vi "Autonomous Independent.vi"   [LabVIEW 2016]
doc: "This VI is called when autonomous begins, and will automatically be terminated when autonomous ends. You can carry out timed or sensor driven robot movement independently without needing to return to the caller."
uses:
  <vilib>/Rock Robotics/WPI/Utilities/WPI_GetSetVariantRefNum.vi
  <vilib>/Rock Robotics/Network Tables/NT Read String.vi
  <vilib>/Rock Robotics/Network Tables/NT Write Numeric Array.vi
  Robot Global Data.vi
  <vilib>/addons/control/pid/pid.llb/PID (DBL).vi
  <vilib>/addons/control/pid/NI_PID_pid.lvlib
panel:
  # "Be sure to right-click and choose Data Operations>>Make Current Value default if you want to save the array values with the VI"
types:
  T1 = typedef "WPI_JoystickDevRef.ctl" = cluster{"Device":T2}
  T2 = typedef "WPI_JoystickDeviceEnum.ctl" = enum16{"USB 0", "USB 1", "USB 2", "USB 3", "USB 4", "USB 5"}
  T3 = typedef "WPI_RobotDriveDevRef.ctl" = cluster{"DevStatus":errorcluster, "Motors[]":T4[], "Square Inputs":bool, "Max Output":dbl}
  T4 = typedef "WPI_MotorControlDeviceRef.ctl" = cluster{"DeviceStatus":errorcluster, "Type":T5, "PWM":cluster{"PWM Channel":T6, "DeadBand":T7}, "CAN":cluster{"Device Number":u8, "SetOutput VI Ref":variant, "GetOutput VI Ref":variant, "Enable VI Ref":variant, "Disable VI Ref":variant, "Data":variant}, "Invert":bool}
  T5 = typedef "WPI_MotorControlType.ctl" = enum16{"PWM", "CAN"}
  T6 = typedef "FPGA_DIOPWMChannel.ctl" = enum8{"PWM 0", "PWM 1", "PWM 2", "PWM 3", "PWM 4", "PWM 5", "PWM 6", "PWM 7", "PWM 8", "PWM 9", "PWM MXP 0", "PWM MXP 1", "PWM MXP 2", "PWM MXP 3", "PWM MXP 4", "PWM MXP 5", "PWM MXP 6", "PWM MXP 7", "PWM MXP 8", "PWM MXP 9", "Invalid"}
  T7 = typedef "WPI_PWMDeadband.ctl" = cluster{"Name":string, "maxPositivePwm":i32, "minPositivePwm":i32, "centerPwm":i32, "maxNegativePwm":i32, "minNegativePwm":i32, "angularRange":u16}
  T8 = cluster{"proportional gain (Kc)":dbl, "integral time (Ti, min)":dbl, "derivative time (Td, min)":dbl}
  T9 = cluster{"Distance (ft)":dbl, "Score":dbl, "Normalized":cluster{"Center":cluster{dbl, dbl}, "Rectangle":cluster{"Numeric":dbl, "Numeric 2":dbl, "Numeric 3":dbl, "Numeric 5":dbl}}, "Pixels":cluster{"Center":cluster{dbl, dbl}, "Rectangle":cluster{"Numeric":dbl, "Numeric 2":dbl, "Numeric 3":dbl, "Numeric 5":dbl}}}
  T10 = cluster{"Yaw":dbl, "Roll":dbl, "Pitch":dbl, "Heading":dbl, "Fused Heading":dbl}
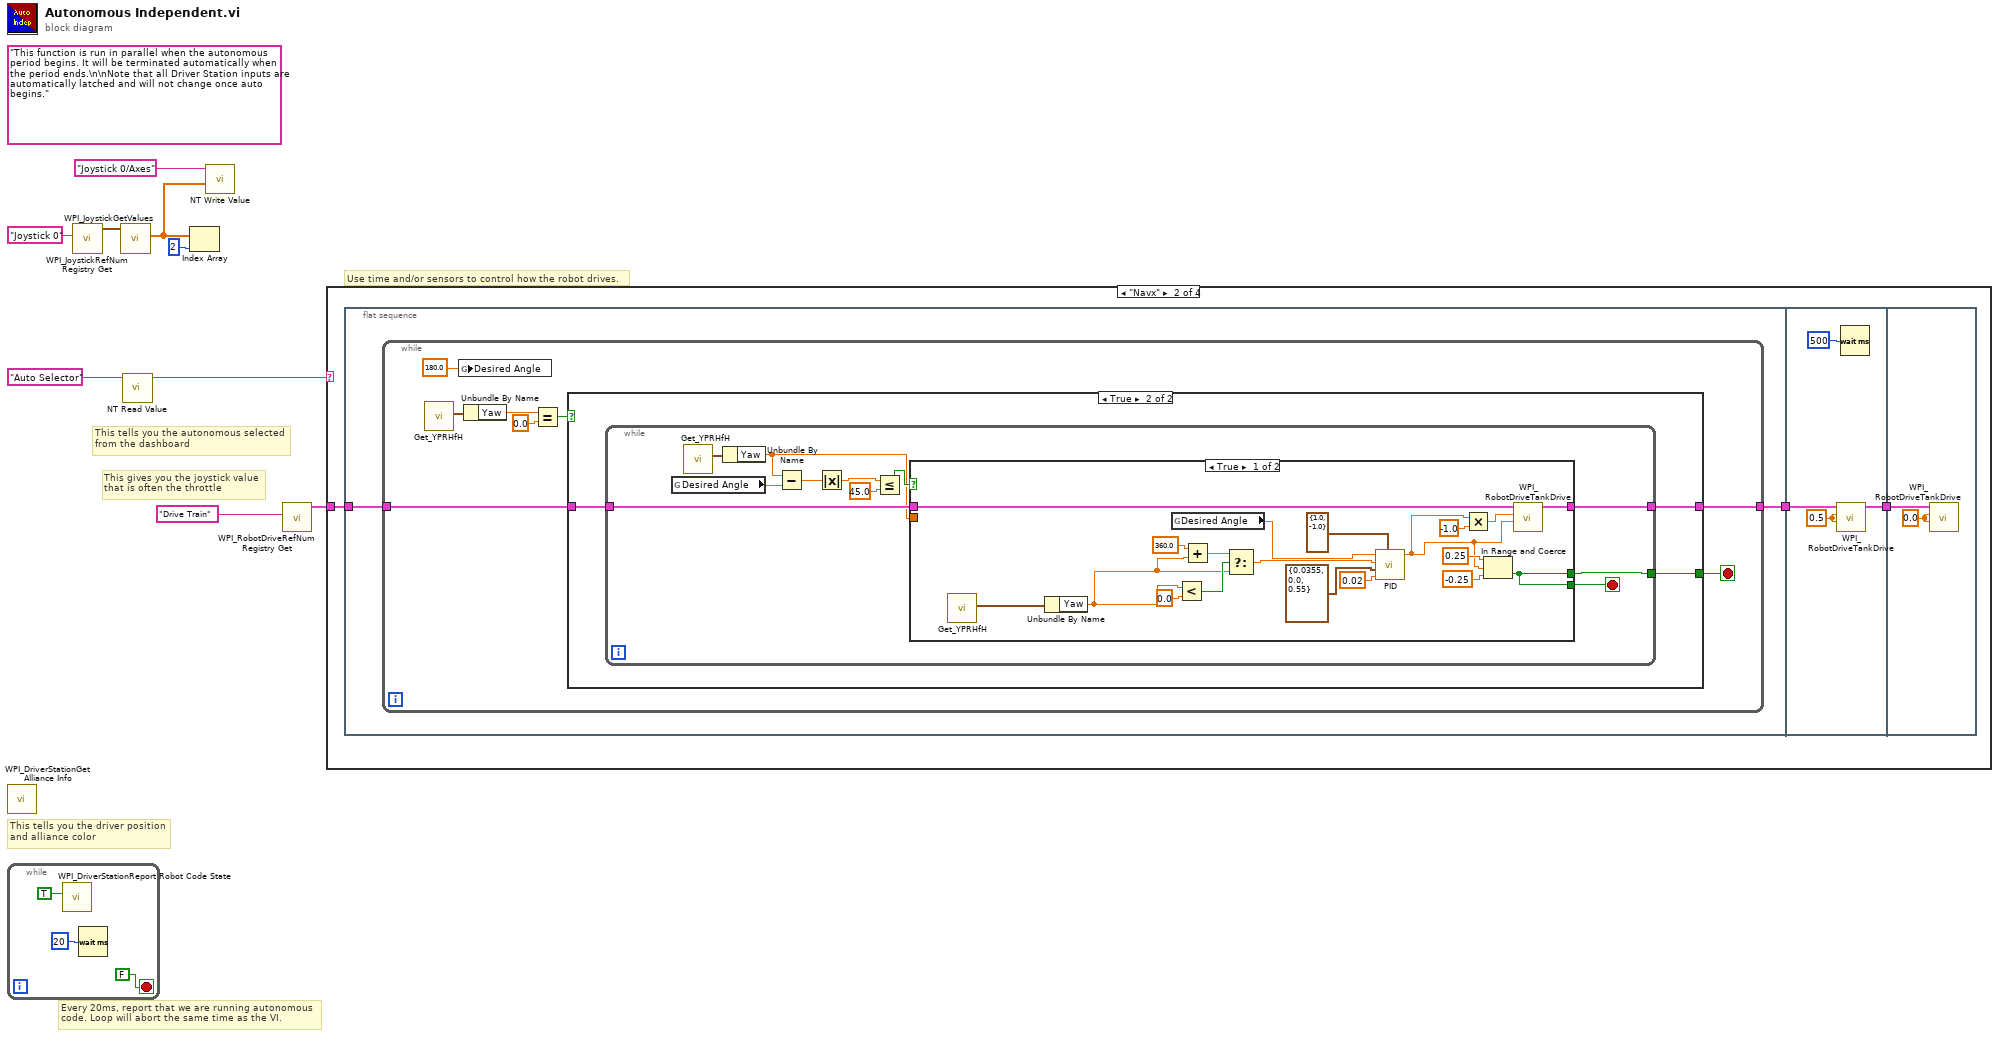
[diagram p0: block diagram]
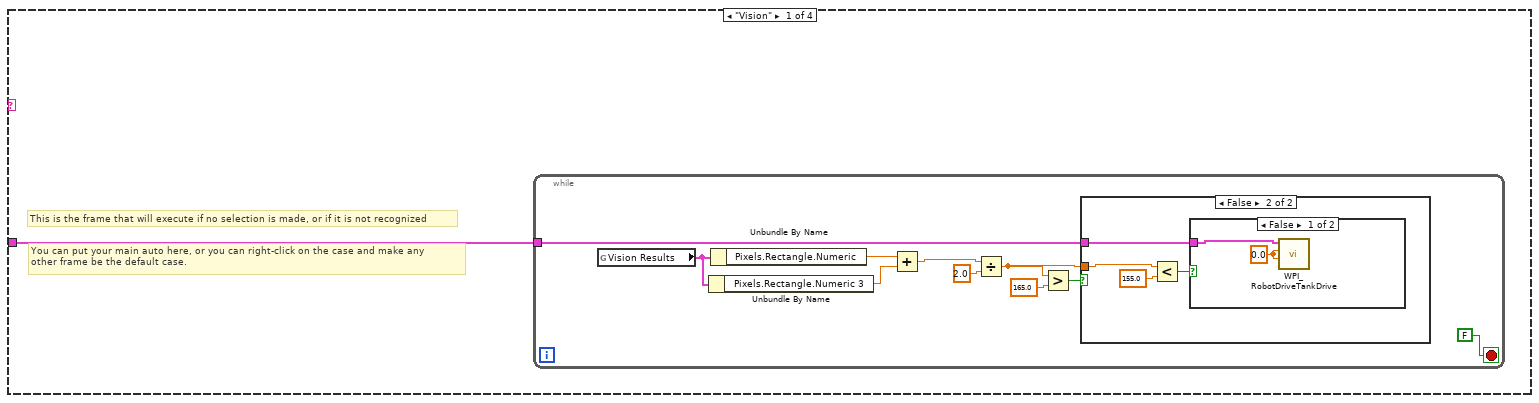
[diagram p2: hidden frame]
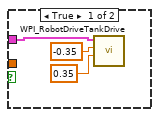
[diagram p3: hidden frame]
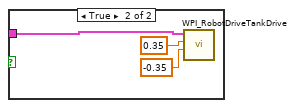
[diagram p4: hidden frame]
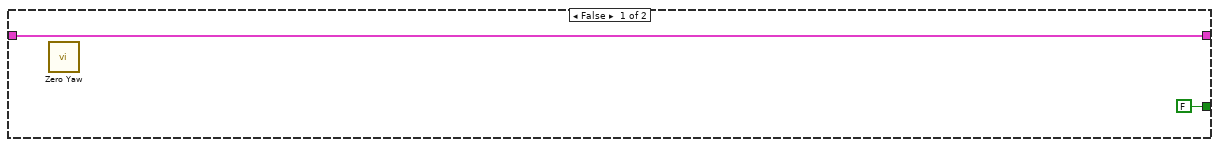
[diagram p5: hidden frame]
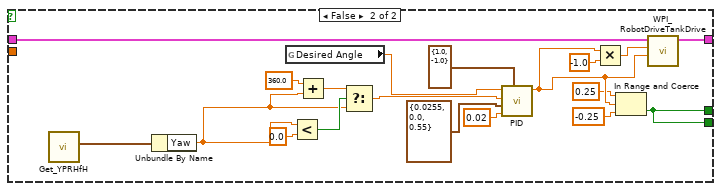
[diagram p6: hidden frame]
diagram:
  (unwired) "This function is run in parallel when the autonomous period begins. It will be terminated automatically when the period ends.\n\nNote that all Driver Station inputs are automatically latched and will not change once auto begins."
  # "This tells you the autonomous selected\nfrom the dashboard"
  # "Every 20ms, report that we are running autonomous\ncode. Loop will abort the same time as the VI."
  # "This gives you the joystick value\nthat is often the throttle"
  # "Use time and/or sensors to control how the robot drives."
  # "This tells you the driver position\nand alliance color"
  n1 = call <vilib>:"WPI_DriverStationGet Alliance Info.vi"() -> ()  [unwired: 12 out]
  n2 = while {
    stop <- FALSE stop-if-true
    n3 = call <vilib>:"WPI_DriverStationReport Robot Code State.vi"("Autonomous"=TRUE) -> ()  [unwired: 10 in, 1 out]
    n4 = Wait (ms)(milliseconds to wait=u32 20) -> ()  [unwired: 1 out]
  }
  n5 = call <vilib>:"WPI_JoystickRefNum Registry Get.vi"("refnum name"="Joystick 0") -> ("JoystickDevRef"=w8:T1)  [unwired: 1 in, 9 out]
  n6 = call <vilib>:"WPI_JoystickGetValues.vi"("JoystickDevRef"=w8) -> ("Axes"=w4:dbl[])  [unwired: 6 in, 4 out]
  n7 = call-poly <vilib>:"NT Read Value.vi"("Name"="Auto Selector") -> ("String"=w5:string)  [unwired: 9 in, 1 out]
  n8 = Index Array(array=w4, index=2) -> ()  [unwired: 1 out]
  n9 = call-poly <vilib>:"NT Write Value.vi"("Numeric Array"=w4, "Name"="Joystick 0/Axes") -> ()  [unwired: 9 in, 1 out]
  n10 = call <vilib>:"WPI_RobotDriveRefNum Registry Get.vi"("refnum name"="Drive Train") -> ("RobotDriveDevRef"=w1:T3)  [unwired: 1 in, 9 out]
  n11 = case shown="\"Navx\"" w5 {
    tunnel: w1 -> [w13 w38 _ _]
    frame "Vision" {
      # "You can put your main auto here, or you can right-click on the case and make any\nother frame be the default case."
      # "This is the frame that will execute if no selection is made, or if it is not recognized"
      n12 = while {
        tunnel: w13 -> [w22]
        stop <- FALSE stop-if-true
        n13 = global read "Robot Global Data.vi" "Vision Results"() -> (w21:T9)
        n14 = Unbundle By Name(w21) -> ("Pixels.Rectangle.Numeric 3"=w19:dbl)
        n15 = Unbundle By Name(w21) -> ("Pixels.Rectangle.Numeric"=w20:dbl)
        n16 = Add(x=w20, y=w19) -> (x+y=w18:dbl)
        n17 = Divide(x=w18, y=2.0) -> (x/y=w16:dbl)
        n18 = Greater?(x=w16, y=165.0) -> (0:w15:bool)
        n19 = case shown="False" w15 {
          tunnel: w22 -> [w26 w30]
          tunnel: w16 -> [_ w27]
          frame True {
            n20 = call <vilib>:"WPI_RobotDriveTankDrive.vi"("Right axis value"=0.35, "Left axis value"=-0.35, "RobotDriveDevRef"=w26) -> ()  [unwired: 6 in, 3 out]
          }
          frame False {
            n21 = Less?(x=w27, y=155.0) -> (x < y?=w28:bool)
            n22 = case shown="False" w28 {
              tunnel: w30 -> [w31 w33]
              frame False {
                w32 = 0.0 ("Left axis value")
                n23 = call <vilib>:"WPI_RobotDriveTankDrive.vi"("Right axis value"=w32, "Left axis value"=w32, "RobotDriveDevRef"=w31) -> ()  [unwired: 6 in, 3 out]
              }
              frame True {
                n24 = call <vilib>:"WPI_RobotDriveTankDrive.vi"("Right axis value"=-0.35, "Left axis value"=0.35, "RobotDriveDevRef"=w33) -> ()  [unwired: 6 in, 3 out]
              }
            }
          }
        }
      }
    }
    frame "Navx" {
      n25 = flat-sequence {
        tunnel: w38 -> [w40]
        tunnel: [w39] -> w37
        tunnel: w37 -> [w106]
        tunnel: [w103] -> w36
        tunnel: w36 -> [w107]
        frame #0 {
          n26 = while {
            tunnel: w40 -> [w48]
            tunnel: [w42] -> w39
            stop <- w41 stop-if-true
            n27 = call <vilib>:"Get_YPRHfH.vi"() -> ("YRPHfH"=w47:T10)  [unwired: 11 in]
            n28 = global write "Robot Global Data.vi" "Desired Angle"(180.0 ("Desired Angle")) -> ()
            n29 = Unbundle By Name(w47) -> ("Yaw"=w46:dbl)
            n30 = Equal?(x=w46, y=0.0) -> (x = y?=w44:bool)
            n31 = case shown="True" w44 {
              tunnel: w48 -> [w50 w53]
              tunnel: [w50 w52] -> w42
              tunnel: [FALSE w51] -> w41
              frame False {
                n32 = call <vilib>:"Zero Yaw.vi"() -> ()  [unwired: 12 in]
              }
              frame True {
                n33 = while {
                  tunnel: w53 -> [w64]
                  tunnel: [w57] -> w52
                  tunnel: [w54] -> w51
                  stop <- w55 stop-if-true
                  n34 = global read "Robot Global Data.vi" "Desired Angle"() -> (w58:dbl)
                  n35 = call <vilib>:"Get_YPRHfH.vi"() -> ("YRPHfH"=w63:T10)  [unwired: 11 in]
                  n36 = Unbundle By Name(w63) -> ("Yaw"=w56:dbl)
                  n37 = Subtract(x=w56, y=w58) -> (x-y=w62:dbl)
                  n38 = Absolute Value(x=w62) -> (abs(x)=w61:dbl)
                  n39 = Less Or Equal?(x=w61, y=45.0) -> (x <= y?=w59:bool)
                  n40 = case shown="True" w59 {
                    tunnel: w64 -> [w79 w98]
                    tunnel: [w69 w89] -> w57
                    tunnel: w56 -> [_ _]
                    tunnel: [w65 w84] -> w55
                    tunnel: [w65 w84] -> w54
                    frame True {
                      n41 = call <vilib>:"Get_YPRHfH.vi"() -> ("YRPHfH"=w83:T10)  [unwired: 11 in]
                      n42 = Unbundle By Name(w83) -> ("Yaw"=w72:dbl)
                      n43 = global read "Robot Global Data.vi" "Desired Angle"() -> (w76:dbl)
                      n44 = Less?(x=w72, y=0.0) -> (x < y?=w73:bool)
                      n45 = Add(x=360.0, y=w72) -> (x+y=w75:dbl)
                      n46 = Select(t=w75, s=w73, f=w72) -> (s? t:f=w71:dbl)
                      n47 = call-poly <vilib>:"PID.vi"("output range"=cluster{"output high":dbl, "output low":dbl} {"output high"=1.0, "output low"=-1.0}, "dt (s)"=0.02, "PID gains"=T8 {"proportional gain (Kc)"=0.0355, "integral time (Ti, min)"=0.0, "derivative time (Td, min)"=0.55}, "process variable"=w71, "setpoint"=w76) -> ("output"=w66:dbl)  [unwired: 5 in, 1 out]
                      n48 = Multiply(x=w66, y=-1.0) -> (x*y=w80:dbl)
                      n49 = In Range and Coerce(upper limit=0.25, x=w66, lower limit=-0.25) -> (In Range?=w65:bool)  [unwired: 1 out]
                      n50 = call <vilib>:"WPI_RobotDriveTankDrive.vi"("Right axis value"=w66, "Left axis value"=w80, "RobotDriveDevRef"=w79) -> ("RobotDriveDevRef"=w69:T3)  [unwired: 6 in, 2 out]
                    }
                    frame False {
                      n51 = call <vilib>:"Get_YPRHfH.vi"() -> ("YRPHfH"=w101:T10)  [unwired: 11 in]
                      n52 = Unbundle By Name(w101) -> ("Yaw"=w88:dbl)
                      n53 = global read "Robot Global Data.vi" "Desired Angle"() -> (w95:dbl)
                      n54 = Less?(x=w88, y=0.0) -> (x < y?=w91:bool)
                      n55 = Add(x=360.0, y=w88) -> (x+y=w94:dbl)
                      n56 = Select(t=w94, s=w91, f=w88) -> (s? t:f=w90:dbl)
                      n57 = call-poly <vilib>:"PID.vi"("output range"=cluster{"output high":dbl, "output low":dbl} {"output high"=1.0, "output low"=-1.0}, "dt (s)"=0.02, "PID gains"=T8 {"proportional gain (Kc)"=0.0255, "integral time (Ti, min)"=0.0, "derivative time (Td, min)"=0.55}, "process variable"=w90, "setpoint"=w95) -> ("output"=w87:dbl)  [unwired: 5 in, 1 out]
                      n58 = Multiply(x=w87, y=-1.0) -> (x*y=w96:dbl)
                      n59 = In Range and Coerce(upper limit=0.25, x=w87, lower limit=-0.25) -> (In Range?=w84:bool)  [unwired: 1 out]
                      n60 = call <vilib>:"WPI_RobotDriveTankDrive.vi"("Right axis value"=w87, "Left axis value"=w96, "RobotDriveDevRef"=w98) -> ("RobotDriveDevRef"=w89:T3)  [unwired: 6 in, 2 out]
                    }
                  }
                }
              }
            }
          }
        }
        frame #1 {
          w105 = 0.5 ("Left axis value")
          n61 = call <vilib>:"WPI_RobotDriveTankDrive.vi"("Right axis value"=w105, "Left axis value"=w105, "RobotDriveDevRef"=w106) -> ("RobotDriveDevRef"=w103:T3)  [unwired: 6 in, 2 out]
          n62 = Wait (ms)(milliseconds to wait=u32 500) -> ()  [unwired: 1 out]
        }
        frame #2 {
          w108 = 0.0 ("Left axis value")
          n63 = call <vilib>:"WPI_RobotDriveTankDrive.vi"("Right axis value"=w108, "Left axis value"=w108, "RobotDriveDevRef"=w107) -> ()  [unwired: 6 in, 3 out]
        }
      }
    }
    frame Default {
    }
    frame "Middle Spring" {
      n64 = flat-sequence {
        frame #0 {
        }
      }
    }
  }
